vi "chartsheet set paper.vi"(8 "error in (no error)":errorcluster, 10 "paper_type":u8, 11 "chartsheet":u32) -> (0 "error out":errorcluster)   [LabVIEW 8.6]
doc: "void chartsheet_set_paper(lxw_chartsheet chartsheet, uint8_t paper_type);"
uses:
  pending_lvxlsxwriter/xlsxwriter.dll
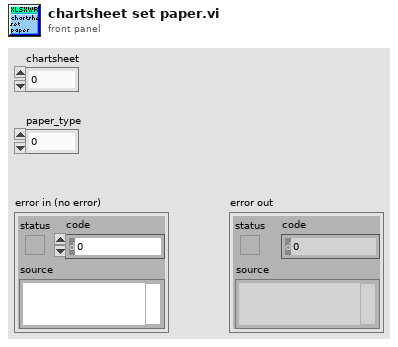
[diagram p1: front panel]
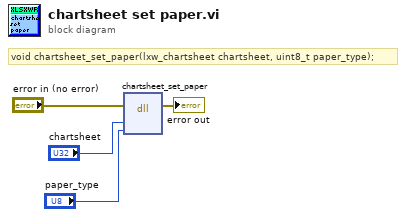
[diagram p0: block diagram]
diagram:
  # "void chartsheet_set_paper(lxw_chartsheet chartsheet, uint8_t paper_type);"
  n1 = dll-call lib="C:/Users/WDAGUtilityAccount/Desktop/pending_lvxlsxwriter/xlsxwriter.*" fn="chartsheet_set_paper"(error in="error in (no error)", "chartsheet"="chartsheet", "paper_type"="paper_type") -> (error out=→"error out":errorcluster)  [unwired: 5 in, 1 out]
